vi "wd_length_replaceAll.vi"(7 "data type":T1=enum."Array of DBL", 8 "error in (no error)":errorcluster, 9 "channel index":u32, 10 "size":u64, 11 "meta in":T2={"TargetFile"=path "", "StreamMode"=enum."File", "Append?"=FALSE, "ChunkSize"=0, "TimeColumnMode"=enum."Empty", "TimestampFormat"="", "AbsoluteTime?"=FALSE, "FileAttribute "={"Creator"="", "Title"="", "SheetName"=""}, "Column"=[], "FileRef"=refnum, "MemoryRef"=[], "RecordInfo"=[], " ChannelPreviousInfo"=[], "ChannelFirstRecord"=[], "PredefinedFormattedValueLength"=20, "DiskTemplate"={"XMLRef"=[refnum, refnum, refnum, refnum, refnum, refnum], "ZipPath"=path "", "MetaFile"={"Ref"=refnum, "NextRow"=0, "NextPosition"=0, "Block"=[]}, "TempFolder"=path ""}}) -> (0 "error out":errorcluster, 3 "meta out":T2={"TargetFile"=path "", "StreamMode"=enum."File", "Append?"=FALSE, "ChunkSize"=0, "TimeColumnMode"=enum."Empty", "TimestampFormat"="", "AbsoluteTime?"=FALSE, "FileAttribute "={"Creator"="", "Title"="", "SheetName"=""}, "Column"=[], "FileRef"=refnum, "MemoryRef"=[], "RecordInfo"=[], " ChannelPreviousInfo"=[], "ChannelFirstRecord"=[], "PredefinedFormattedValueLength"=20, "DiskTemplate"={"XMLRef"=[refnum, refnum, refnum, refnum, refnum, refnum], "ZipPath"=path "", "MetaFile"={"Ref"=refnum, "NextRow"=0, "NextPosition"=0, "Block"=[]}, "TempFolder"=path ""}})   [LabVIEW 2017, in "NI_ExcelFile.lvlib"]
uses:
  <vilib>/express/express shared/NI_ExcelFile/NI_ExcelFile.lvlib
  <vilib>/express/express shared/NI_ExcelFile/Ctrls/MainData.ctl
  <vilib>/express/express shared/NI_ExcelFile/Ctrls/StreamMode.ctl
  <vilib>/express/express shared/NI_ExcelFile/Ctrls/TimeColumnMode.ctl
  <vilib>/express/express shared/NI_ExcelFile/Ctrls/FileAttribute.ctl
  <vilib>/express/express shared/NI_ExcelFile/Ctrls/Columns.ctl
  <vilib>/express/express shared/NI_ExcelFile/Ctrls/ColumnInfo.ctl
  <vilib>/express/express shared/NI_ExcelFile/Ctrls/DataType.ctl
  <vilib>/express/express shared/NI_ExcelFile/Ctrls/wd_recordInfo.ctl
  <vilib>/express/express shared/NI_ExcelFile/Ctrls/disk_TemplateFile.ctl
  <vilib>/express/express shared/NI_ExcelFile/Ctrls/meta_file.ctl
  <vilib>/express/express shared/NI_ExcelFile/Ctrls/meta_Block.ctl
  <vilib>/express/express shared/NI_ExcelFile/Ctrls/meta_BlockType.ctl
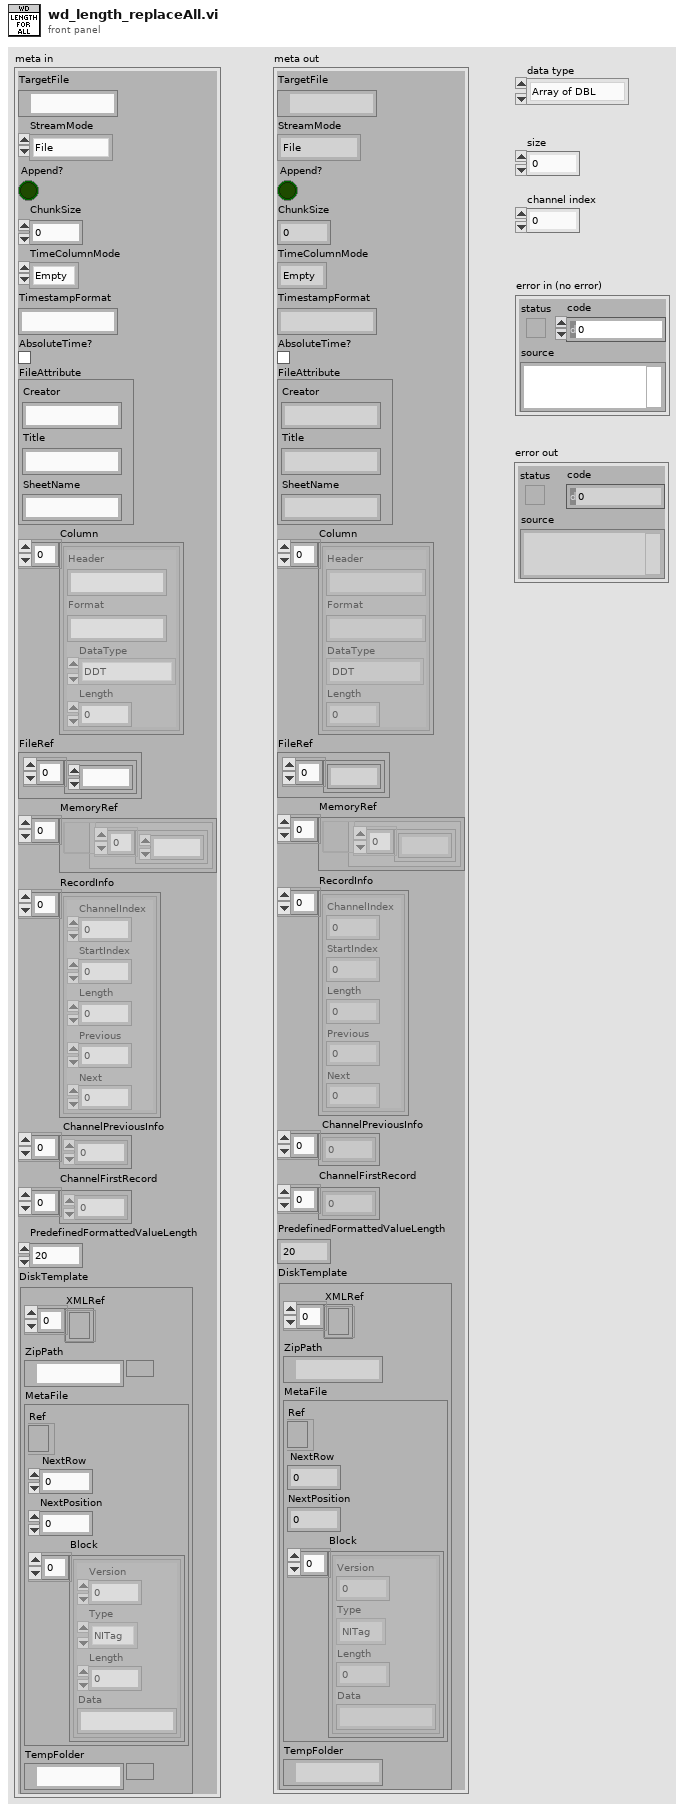
[diagram p1: front panel]
types:
  T1 = typedef "NI_ExcelFile.lvlib/DataType.ctl" = enum16{"DDT", "WFM", "Array of STR", "Array of DBL", "Array of I8", "Array of I16", "Array of I32", "Array of I64", "Array of SGL", "Array of U8", "Array of U16", "Array of U32", "Array of U64", "Array of Time"}
  T2 = typedef "NI_ExcelFile.lvlib/MainData.ctl" = cluster{"TargetFile":path, "StreamMode":T3, "Append?":bool, "ChunkSize":u64, "TimeColumnMode":T4, "TimestampFormat":string, "AbsoluteTime?":bool, "FileAttribute ":T5, "Column":T6, "FileRef":refnum<k1>, "MemoryRef":refnum<data-value>[], "RecordInfo":T8[], " ChannelPreviousInfo":u32[], "ChannelFirstRecord":u32[], "PredefinedFormattedValueLength":i64, "DiskTemplate":T9}
  T3 = typedef "NI_ExcelFile.lvlib/StreamMode.ctl" = enum16{"File", "Memory"}
  T4 = typedef "NI_ExcelFile.lvlib/TimeColumnMode.ctl" = enum16{"Empty", "OnePerCh", "One"}
  T5 = typedef "NI_ExcelFile.lvlib/FileAttribute.ctl" = cluster{"Creator":string, "Title":string, "SheetName":string}
  T6 = typedef "NI_ExcelFile.lvlib/Columns.ctl" = T7[]
  T7 = typedef "NI_ExcelFile.lvlib/ColumnInfo.ctl" = cluster{"Header":string, "Format":string, "DataType":T1, "Length":u64}
  T8 = typedef "NI_ExcelFile.lvlib/wd_recordInfo.ctl" = cluster{"ChannelIndex":u32, "StartIndex":u64, "Length":u64, "Previous":i32, "Next":i32}
  T9 = typedef "NI_ExcelFile.lvlib/disk_TemplateFile.ctl" = cluster{"XMLRef":refnum<file>[], "ZipPath":path, "MetaFile":T10, "TempFolder":path}
  T10 = typedef "NI_ExcelFile.lvlib/meta_file.ctl" = cluster{"Ref":refnum<file>, "NextRow":i32, "NextPosition":i64, "Block":T11[]}
  T11 = typedef "NI_ExcelFile.lvlib/meta_Block.ctl" = cluster{"Version":u16, "Type":T12, "Length":i32, "Data":string}
  T12 = typedef "NI_ExcelFile.lvlib/meta_BlockType.ctl" = enum16{"NITag", "File", "Column"}
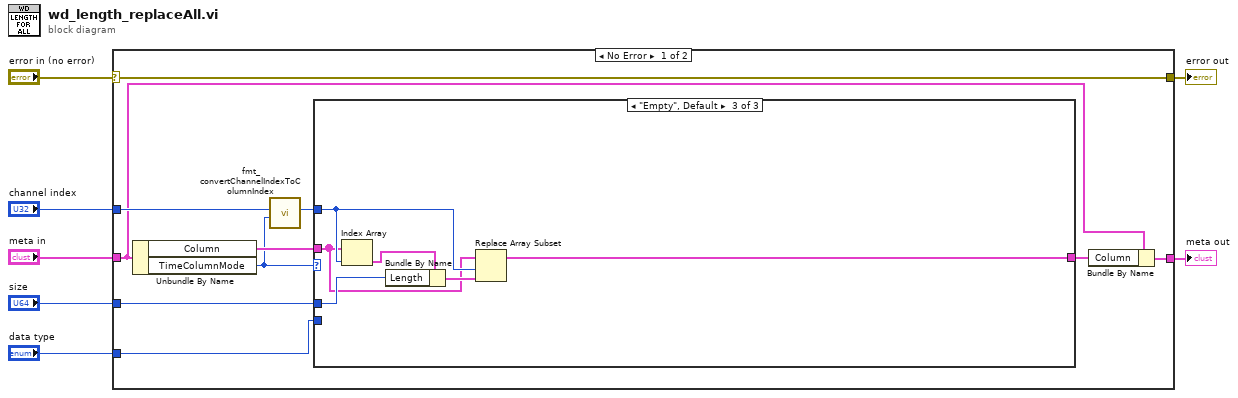
[diagram p0: block diagram]
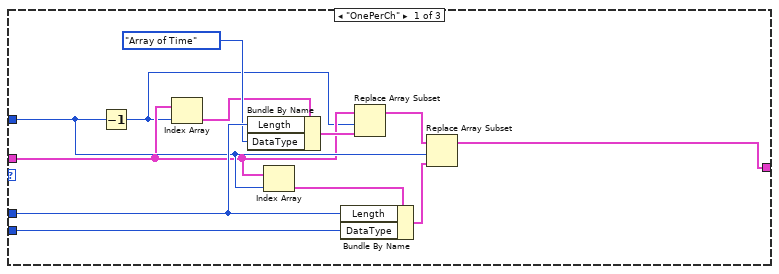
[diagram p2: hidden frame]
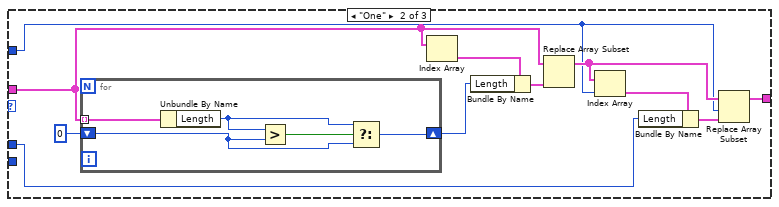
[diagram p3: hidden frame]
diagram:
  n1 = case shown="No Error" "error in (no error)" {
    selector: "error in (no error)" -> [w8 w52]
    tunnel: [w17 w53] -> w7
    tunnel: "meta in" -> [w9 w53]
    tunnel: "size" -> [w15 _]
    tunnel: "channel index" -> [w12 _]
    tunnel: "data type" -> [w13 _]
    tunnel: [w8 w52] -> w1
    frame No Error {
      n2 = Unbundle By Name(w9) -> ("Column"=w14:T6, "TimeColumnMode"=w11:T4)
      n3 = call <vilib>:"fmt_convertChannelIndexToColumnIndex.vi"("TimeColumnMode"=w11, "channel index"=w12) -> ("data column index"=w10:i32)  [unwired: 8 in, 1 out]
      n4 = case shown="\"Empty\", Default" w11 {
        tunnel: w14 -> [w20 w36 w47]
        tunnel: [w25 w30 w46] -> w16
        tunnel: w10 -> [w21 w32 w49]
        tunnel: w15 -> [w28 w34 w50]
        tunnel: w13 -> [w23 _ _]
        frame "OnePerCh" {
          n5 = Decrement(x=w21) -> (x-1=w19:i32)
          n6 = Index Array(array=w20, index=w19) -> (element=w18:T7)
          n7 = Bundle By Name(cluster=w18, "Length"=w28, "DataType"=DataType."Array of Time" ("Column DataType")) -> (w29:T7)
          n8 = Index Array(array=w20, index=w21) -> (element=w22:T7)
          n9 = Bundle By Name(cluster=w22, "Length"=w28, "DataType"=w23) -> (w26:T7)
          n10 = Replace Array Subset(array=w20, new element=w29, index=w19) -> (w27:T6)
          n11 = Replace Array Subset(array=w27, new element=w26, index=w21) -> (w25:T6)
        }
        frame "One" {
          n12 = for {
            tunnel: w36 -> [w45] mode=indexing
            shift-right: [w41] -> w39
            shift-left: u64 0 -> [w42]
            n13 = Unbundle By Name(w45) -> ("Length"=w43:u64)
            n14 = Greater?(x=w43, y=w42) -> (0:w44:bool)
            n15 = Select(t=w43, s=w44, f=w42) -> (s? t:f=w41:u64)
          }
          n16 = Index Array(array=w36) -> (element=w38:T7)  [unwired: 1 in]
          n17 = Bundle By Name(cluster=w38, "Length"=w39) -> (w37:T7)
          n18 = Replace Array Subset(array=w36, new element=w37) -> (w33:T6)  [unwired: 1 in]
          n19 = Index Array(array=w33, index=w32) -> (element=w35:T7)
          n20 = Bundle By Name(cluster=w35, "Length"=w34) -> (w31:T7)
          n21 = Replace Array Subset(array=w33, new element=w31, index=w32) -> (w30:T6)
        }
        frame "Empty", Default {
          n22 = Index Array(array=w47, index=w49) -> (element=w51:T7)
          n23 = Bundle By Name(cluster=w51, "Length"=w50) -> (w48:T7)
          n24 = Replace Array Subset(array=w47, new element=w48, index=w49) -> (w46:T6)
        }
      }
      n25 = Bundle By Name(cluster=w9, "Column"=w16) -> (w17:T2)
    }
    frame Error {
    }
  }
  "meta out" <- w7
  "error out" <- w1
